vi "Start.vi"(8 "Error In":errorcluster, 11 "reference in":refnum<class "Thermometer Multichannel.lvclass">) -> (0 "Error Out":errorcluster, 3 "reference out":refnum<class "Thermometer Multichannel.lvclass">)   [LabVIEW 2024, in "Thermometer Multichannel.lvclass"]
uses:
  Thermometer Multichannel.lvclass
  Interfaces/IRunnable/IRunnable.lvclass
  Thermometer Multichannel Worker/Thermometer Multichannel Worker/Thermometer Multichannel Worker.lvclass
  Interfaces/IRead Temperature Multichannel/IRead Temperature Multichannel.lvclass
  <vilib>/ActorFramework/Actor/Actor.lvclass
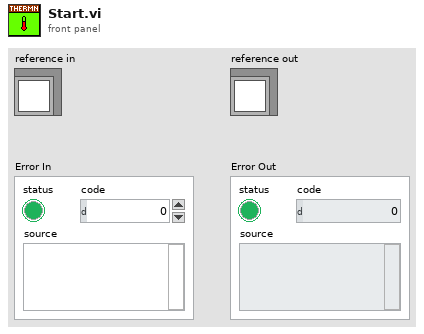
[diagram p1: front panel]
types:
  T1 = typedef "Thermometer Multichannel.lvclass/ObjectAttributes.ctl" = cluster{"IConfigure":refnum<class "IConfigure.lvclass">, "Worker Enqueuer":refnum<class "Message Enqueuer.lvclass">}
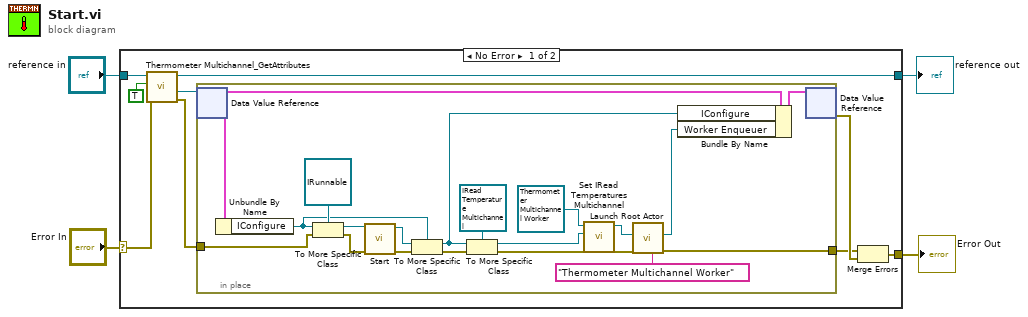
[diagram p0: block diagram]
diagram:
  n1 = case shown="No Error" "Error In" {
    selector: "Error In" -> [w13 w34]
    tunnel: [w7 w34] -> w3
    tunnel: [w11 w33] -> w1
    tunnel: "reference in" -> [w12 w33]
    frame No Error {
      n2 = call "Thermometer Multichannel_GetAttributes.vi"("Error In"=w13, "OnlyGetDvrReference(False)"=TRUE, "reference in"=w12) -> ("Error Out"=w8:errorcluster, "DataRef"=w9:refnum<data-value>, "reference out"=w11:refnum<class "Thermometer Multichannel.lvclass">)  [unwired: 5 in, 1 out]
      n3 = in-place {
        in-place-border: w8 -> [w26]
        in-place-border: [w25] -> w5
        n4 = in-place-dvr #1(w9) -> (w31:T1)  [unwired: 1 out]
        n5 = Unbundle By Name(w31) -> ("IConfigure"=w18:refnum<class "IConfigure.lvclass">)
        n6 = To More Specific Class(target class=refnum<class "IRunnable.lvclass"> refnum ("IRunnable.lvclass"), reference=w18, error in=w26) -> (specific class reference=w29:refnum<class "IRunnable.lvclass">, error out=w28:errorcluster)
        n7 = call-dynamic "Start.vi"("error in"=w28, "IRunnable in"=w29) -> ("error out"=w27:errorcluster, "IRunnable out"=w19:refnum<class "IRunnable.lvclass">)  [unwired: 8 in]
        n8 = To More Specific Class(target class=w18, reference=w19, error in=w27) -> (specific class reference=w17:refnum<class "IConfigure.lvclass">, error out=w20:errorcluster)
        n9 = To More Specific Class(target class=refnum<class "IRead Temperature Multichannel.lvclass"> refnum ("IRead Temperature Multichannel.lvclass"), reference=w17, error in=w20) -> (specific class reference=w16:refnum<class "IRead Temperature Multichannel.lvclass">, error out=w14:errorcluster)
        n10 = call "Set IRead Temperatures Multichannel.vi"("IRead Temperatures Multichannel"=w16, "Thermometer Multichannel Worker in"=refnum<class "Thermometer Multichannel Worker.lvclass"> refnum ("Communicator Worker.lvlib:Worker.lvclass")) -> ("Thermometer Multichannel Worker out"=w15:refnum<class "Thermometer Multichannel Worker.lvclass">)  [unwired: 9 in]
        n11 = call <vilib>:"Launch Root Actor.vi"("Debug Alias"="Thermometer Multichannel Worker", "error in (no error)"=w14, "Actor"=w15) -> ("error out"=w25:errorcluster, "Actor's Enqueuer"=w23:refnum<class "Message Enqueuer.lvclass">)  [unwired: 7 in]
        n12 = Bundle By Name(cluster=w31, "IConfigure"=w17, "Worker Enqueuer"=w23) -> (w32:T1)
        n13 = in-place-dvr #1(w32) -> (w6:errorcluster)  [unwired: 1 out]
      }
      n14 = Merge Errors(w5, w6) -> (w7:errorcluster)
    }
    frame Error {
    }
  }
  "Error Out" <- w3
  "reference out" <- w1
